vi "MINST_1D_to_mutiplicate_2D_sub.vi"(0 "pattern 1D":i32[](array[numeric]), 1 "No.Multi":i32) -> (2 "Multiplicated_2D":i32[][](array[numeric]), 3 "Pattern_Y":i16=9, 4 "PatternOut":i32[](array[numeric]))   [LabVIEW 2021]
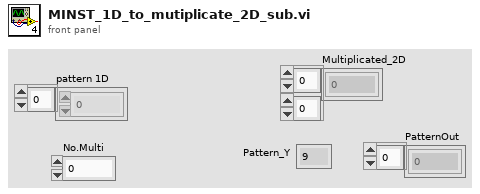
[diagram p1: front panel]
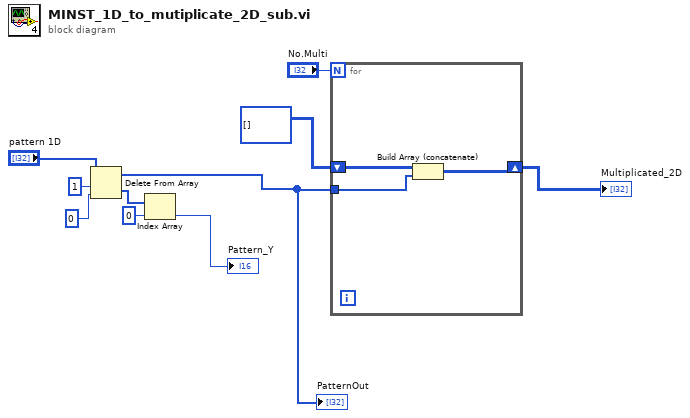
[diagram p0: block diagram]
diagram:
  n1 = Delete From Array(array="pattern 1D", length=1, index=0) -> (deleted portion=w8:i32[], array with subset deleted=w1:i32[])
  "PatternOut" <- w1
  n2 = Index Array(array=w8, index=0) -> (element=→"Pattern_Y":i32)
  n3 = for {
    N: "No.Multi" -> [_]
    shift-right: [w13] -> w2
    shift-left: i32[][] [] -> [w12]
    tunnel: w1 -> [w11]
    n4 = Build Array (concatenate)(w12, w11) -> (w13:i32[][])
  }
  "Multiplicated_2D" <- w2
